vi "Send-to-self.vi"(8 "error in (no error)":errorcluster, 11 "Client in":T1) -> (0 "error out":errorcluster, 3 "Client out":T1)   [LabVIEW 2013, in "PowderDeposition.lvlib" / "PD-Client.lvclass"]
doc: "Send a message to the specified list of receivers.\nThe message is added to the back of the server message queue for processing.\nThe message needs to be created beforehand, either manually or through the 'Create-message' function and any specific contents need to be pre-configured. This function takes care of the sender and time information.\nThe receivers must be provided as an array. Each receiver entry can be composed in two ways: either '<module type>' to send to all active clients of the specified type, or '<module type><module ID>' to send to a specific client. Optionally the special client types 'All' or 'Server' can be used to send the message to all active clients (server excluded) or to the server, respectively."
uses:
  PD-Client.lvclass
  Object-reference.ctl
  PD-Client.lvclass/PD-Client.ctl
  Main/PD-Main.lvclass
  SA-SLMAPI/Sources/Heartbeat/Heartbeat.lvclass
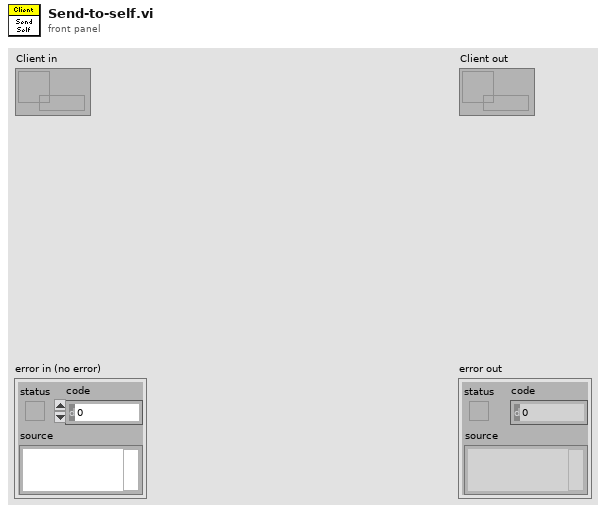
[diagram p1: front panel]
types:
  T1 = typedef "PowderDeposition.lvlib/PD-Client.lvclass/Object-reference.ctl" = refnum<data-value>
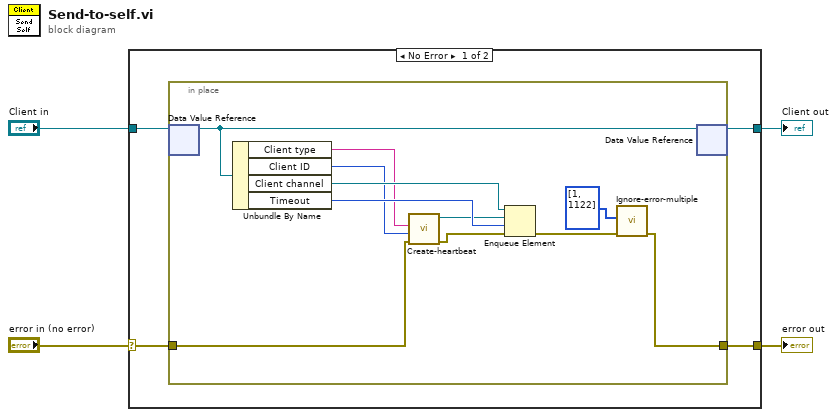
[diagram p0: block diagram]
diagram:
  n1 = case shown="No Error" "error in (no error)" {
    selector: "error in (no error)" -> [w6 w21]
    tunnel: [w5 w21] -> w3
    tunnel: [w7 w20] -> w1
    tunnel: "Client in" -> [w8 w20]
    frame No Error {
      n2 = in-place {
        in-place-border: w6 -> [w10]
        in-place-border: [w15] -> w5
        n3 = in-place-dvr #1(w8) -> (w9:refnum<class "PD-Client.lvclass">)  [unwired: 1 out]
        n4 = Unbundle By Name(w9) -> ("Client type"=w11:string, "Client ID"=w12:i32, "Client channel"=w18:refnum<queue>, "Timeout"=w19:i32)
        n5 = call "Create-heartbeat.vi"("error in (no error)"=w10, "Sender ID"=w12, "Sender"=w11) -> ("error out"=w13:errorcluster, "Heartbeat out"=w14:refnum<class "Heartbeat.lvclass">)  [unwired: 7 in]
        n6 = Enqueue Element(queue=w18, element=w14, timeout in ms (-1)=w19, error in (no error)=w13) -> (error out=w17:errorcluster)  [unwired: 2 out]
        n7 = call "Ignore-error-multiple.vi"("error in (no error)"=w17, "Errors to ignore (1)"=i32[] [1, 1122]) -> ("error out"=w15:errorcluster)  [unwired: 9 in]
        n8 = in-place-dvr #1(w9) -> (w7:T1)  [unwired: 1 out]
      }
    }
    frame Error {
    }
  }
  "error out" <- w3
  "Client out" <- w1
